vi "JSON to Map.vi"(6 "LVClass Serializer":refnum<class "JSONtext LVClass Serializer.lvclass">, 8 "error in (no error)":errorcluster, 9 "Map Type in":variant, 10 "Offset":i32, 11 "<JSON>":string) -> (0 "error out":errorcluster, 1 "Map":variant)   [LabVIEW 2024, in "JSONtext.lvlib" / "SetMap.lvlib"]
uses:
  SetMap.lvlib
  JSONtext LVClass Serializer.lvclass
  SubType.vi
  NI_Data Type.lvlib
  JSONtext.lvlib
  JDP Utility.lvlib
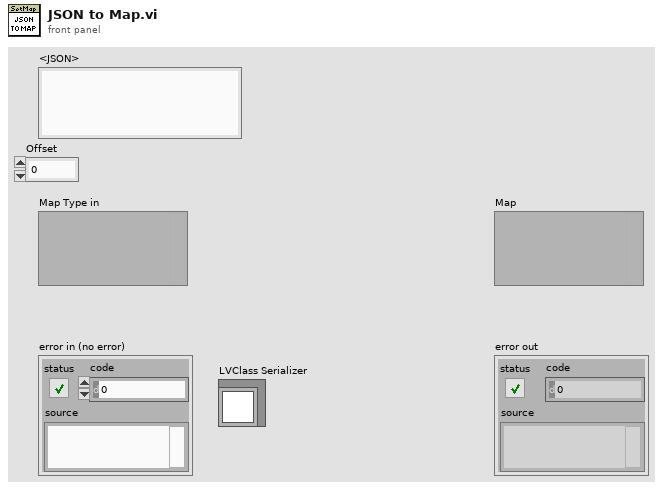
[diagram p1: front panel]
types:
  T1 = typedef "JSONtext.lvlib/JSON Value Type.ctl" = enum16{"Not a JSON Value", "JSON Object", "JSON Array", "String", "Number", "true", "false", "null"}
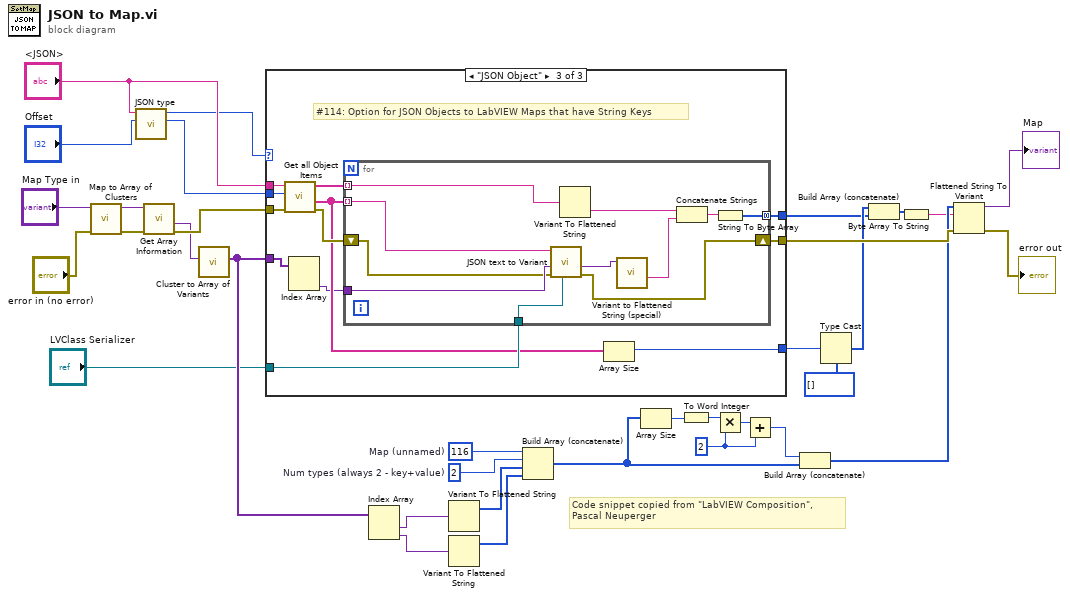
[diagram p0: block diagram]
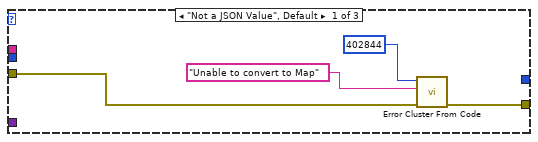
[diagram p2: hidden frame]
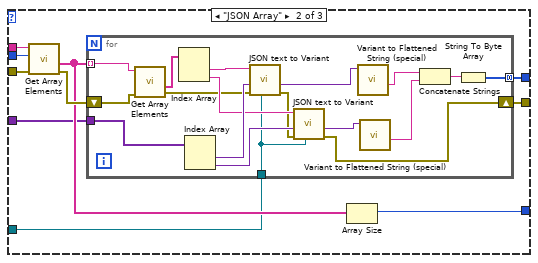
[diagram p3: hidden frame]
diagram:
  w17 = i16 2 ("x")
  w11 = i16 2  # Num types (always 2 - key+value)
  w10 = i16 116  # Map (unnamed)
  # "Code snippet copied from \"LabVIEW Composition\",\nPascal Neuperger"
  n1 = call "Map to Array of Clusters.vi"("error in"="error in (no error)", "Map"="Map Type in") -> ("error out"=w30:errorcluster, "Array of Clusters (key-value)"=w6:variant)  [unwired: 8 in]
  n2 = call "JSON type.vi"("Offset"="Offset", "JSON"="<JSON>") -> ("Item Offset"=w2:i32, "JSON Value Type"=w1:T1)  [unwired: 8 in]
  n3 = call "Get Array Information.vi"("error in (no error)"=w30, "variant"=w6) -> ("error out"=w31:errorcluster, "array element data type"=w7:variant)  [unwired: 6 in, 2 out]
  n4 = call "Cluster to Array of Variants.vi"("Cluster"=w7) -> ("Array of Cluster Elements"=w18:variant[])  [unwired: 10 in]
  n5 = case shown="\"JSON Object\"" w1 {
    tunnel: [w38 w48 w78] -> w32
    tunnel: w31 -> [w37 w46 w73]
    tunnel: [_ w44 w77] -> w25
    tunnel: [_ w43 w76] -> w21
    tunnel: w18 -> [_ w42 w69]
    tunnel: "LVClass Serializer" -> [_ w41 w75]
    tunnel: w2 -> [_ w40 w72]
    tunnel: "<JSON>" -> [_ w39 w74]
    frame "Not a JSON Value", Default {
      n6 = call "Error Cluster From Code.vi"("error in (no error)"=w37, "error message (\"\")"="Unable to convert to Map" ("error message (\"\")"), "error code (402840+)"=402844) -> ("error out"=w38:errorcluster)  [unwired: 6 in]
    }
    frame "JSON Array" {
      n7 = call "Get Array Elements.vi"("error in (no error)"=w46, "Offset"=w40, "JSON"=w39) -> ("error out"=w47:errorcluster, "<JSON>"=w45:string[])  [unwired: 6 in, 1 out]
      n8 = for {
        tunnel: w45 -> [w66] mode=indexing
        tunnel: w42 -> [w63]
        tunnel: [w56] -> w43 mode=concatenating
        shift-right: [w52] -> w48
        shift-left: w47 -> [w55]
        tunnel: w41 -> [w51]
        n9 = call "Get Array Elements.vi"("error in (no error)"=w55, "JSON"=w66) -> ("error out"=w54:errorcluster, "<JSON>"=w65:string[])  [unwired: 7 in, 1 out]
        n10 = Index Array(array=w65) -> (element #1=w64:string, element #2=w61:string)  [unwired: 2 in]
        n11 = Index Array(array=w63) -> (element #1=w62:variant, element #2=w60:variant)  [unwired: 2 in]
        n12 = call "JSON text to Variant.vi"("LVClass Serializer"=w51, "error in (no error)"=w54, "Data Type"=w62, "JSON"=w64) -> ("error out"=w53:errorcluster, "Variant out"=w49:variant)  [unwired: 6 in]
        n13 = call "JSON text to Variant.vi"("LVClass Serializer"=w51, "error in (no error)"=w53, "Data Type"=w60, "JSON"=w61) -> ("error out"=w52:errorcluster, "Variant out"=w50:variant)  [unwired: 6 in]
        n14 = call "Variant to Flattened String (special).vi"("Variant"=w49) -> ("data"=w59:string)  [unwired: 9 in, 1 out]
        n15 = call "Variant to Flattened String (special).vi"("Variant"=w50) -> ("data"=w58:string)  [unwired: 9 in, 1 out]
        n16 = Concatenate Strings(w59, w58) -> (w57:string)
        n17 = String To Byte Array(string=w57) -> (unsigned byte array=w56:u8[])
      }
      n18 = Array Size(array=w45) -> (size(s)=w44:i32)
    }
    frame "JSON Object" {
      # "#114: Option for JSON Objects to LabVIEW Maps that have String Keys"
      n19 = call "Get all Object Items.vi"("error in (no error)"=w73, "Offset"=w72, "JSON"=w74) -> ("error out"=w71:errorcluster, "<JSON>"=w70:string[], "Item Names"=w67:string[])  [unwired: 5 in, 1 out]
      n20 = Index Array(array=w69) -> (element #2=w68:variant)  [unwired: 2 in, 1 out]
      n21 = for {
        tunnel: w70 -> [w82] mode=indexing
        tunnel: [w87] -> w76 mode=concatenating
        shift-right: [w86] -> w78
        shift-left: w71 -> [w81]
        tunnel: w75 -> [w85]
        tunnel: w68 -> [w83]
        tunnel: w67 -> [w80] mode=indexing
        n22 = call "JSON text to Variant.vi"("LVClass Serializer"=w85, "error in (no error)"=w81, "Data Type"=w83, "JSON"=w82) -> ("error out"=w86:errorcluster, "Variant out"=w84:variant)  [unwired: 6 in]
        n23 = Variant To Flattened String(Variant=w80) -> (data string=w79:string)  [unwired: 1 out]
        n24 = call "Variant to Flattened String (special).vi"("Variant"=w84) -> ("data"=w89:string)  [unwired: 9 in, 1 out]
        n25 = Concatenate Strings(w79, w89) -> (w88:string)
        n26 = String To Byte Array(string=w88) -> (unsigned byte array=w87:u8[])
      }
      n27 = Array Size(array=w70) -> (size(s)=w77:i32)
    }
  }
  n28 = Index Array(array=w18) -> (element #1=w19:variant, element #2=w20:variant)  [unwired: 2 in]
  n29 = Variant To Flattened String(Variant=w19) -> (1:w8:i16[])  [unwired: 1 out]
  n30 = Variant To Flattened String(Variant=w20) -> (1:w9:i16[])  [unwired: 1 out]
  n31 = Build Array (concatenate)(w10, w11, w8, w9) -> (w13:i16[])
  n32 = Array Size(array=w13) -> (size(s)=w12:i32)
  n33 = To Word Integer(number=w12) -> (16bit integer=w14:i16)
  n34 = Multiply(x=w14, y=w17) -> (x*y=w15:i16)
  n35 = Add(x=w15, y=w17) -> (x+y=w16:i16)
  n36 = Build Array (concatenate)(w16, w13) -> (w23:i16[])
  n37 = Type Cast(type=u8[] [], x=w25) -> (*(type *) &x=w28:u8[])
  n38 = Build Array (concatenate)(w28, w21) -> (w27:u8[])
  n39 = Byte Array To String(unsigned byte array=w27) -> (string=w22:string)
  n40 = Flattened String To Variant(4:w32, 6:w22, 7:w23) -> (0:→"error out":errorcluster, 3:→"Map":variant)
